vi "g_Identifiers.vi"() -> ()   [LabVIEW 2023, in "Main.lvlib" / "Main.lvclass"]
uses:
  Project/Main.lvclass
panel:
  in  "Report Viewer":string="ReportView"
  in  "Report Generator":string="ReportGen"
  in  "Chronometer":string="Chronometer"
  in  "Debugger":string="Debug"
  in  "Automation":string="Automation"
  in  "Configuration":string="Config"
  in  "Fault Monitor":string="Fault_Mon"
  in  "Manual Buttons":string="M_Butt"
  in  "Manual UI":string="Manual"
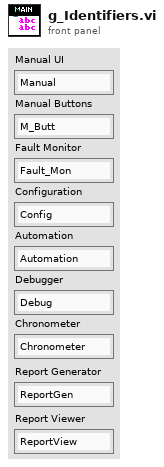
[diagram p1: front panel]
diagram:
